vi "dummy VI.vi"   [LabVIEW 2020]
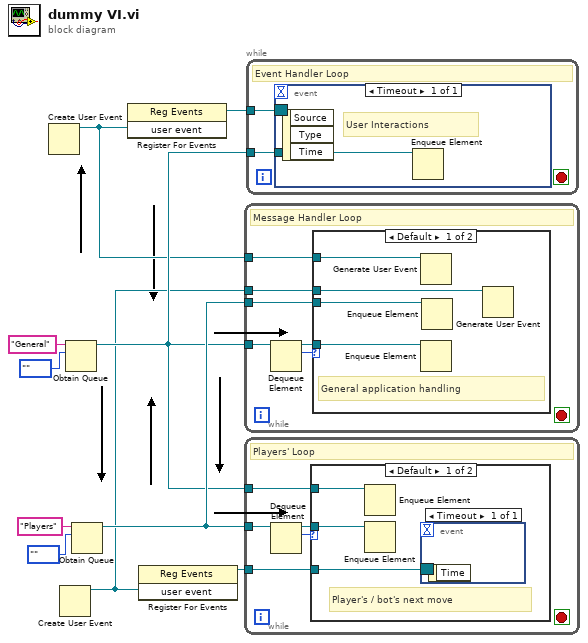
[diagram p0: block diagram]
diagram:
  n1 = Create User Event() -> (user event=w3:refnum<user-event>)  [unwired: 2 in, 1 out]
  n2 = Create User Event() -> (user event=w1:refnum<user-event>)  [unwired: 2 in, 1 out]
  n3 = Obtain Queue(name (unnamed)="General", element data type=enum16{""}."") -> (queue out=w7:refnum<queue>)  [unwired: 3 in, 2 out]
  n4 = Obtain Queue(name (unnamed)="Players", element data type=enum16{""}."") -> (queue out=w8:refnum<queue>)  [unwired: 3 in, 2 out]
  n5 = register-events(w3) -> (reference out=w4:refnum<event-registration>)  [unwired: 2 in, 1 out]
  n6 = register-events(w1) -> (reference out=w2:refnum<event-registration>)  [unwired: 2 in, 1 out]
  n7 = while {
    tunnel: w7 -> [w16]
    tunnel: w8 -> [w13]
    tunnel: w3 -> [w12]
    tunnel: w1 -> [w11]
    stop <- _ stop-if-true
    # "Message Handler Loop"
    n8 = Dequeue Element(queue=w16) -> (queue out=w14:refnum<queue>, element=w15:enum16{""})  [unwired: 2 in, 2 out]
    n9 = case shown="Default" w15 {
      tunnel: w14 -> [w20 _]
      tunnel: w13 -> [w19 _]
      tunnel: w12 -> [w18 _]
      tunnel: w11 -> [w17 _]
      frame Default {
        # "General application handling"
        n10 = Generate User Event(user event=w18) -> ()  [unwired: 3 in, 2 out]
        n11 = Enqueue Element(queue=w20) -> ()  [unwired: 3 in, 3 out]
        n12 = Enqueue Element(queue=w19) -> ()  [unwired: 3 in, 3 out]
        n13 = Generate User Event(user event=w17) -> ()  [unwired: 3 in, 2 out]
      }
      frame "" {
      }
    }
  }
  n14 = while {
    tunnel: w7 -> [w22]
    tunnel: w8 -> [w25]
    tunnel: w2 -> [w21]
    stop <- _ stop-if-true
    # "Players' Loop"
    n15 = Dequeue Element(queue=w25) -> (queue out=w23:refnum<queue>, element=w24:enum16{""})  [unwired: 2 in, 2 out]
    n16 = case shown="Default" w24 {
      tunnel: w23 -> [w27 _]
      tunnel: w22 -> [w28 _]
      tunnel: w21 -> [w26 _]
      frame #0 {
        # "Player's / bot's next move"
        n17 = Enqueue Element(queue=w28) -> ()  [unwired: 3 in, 3 out]
        n18 = Enqueue Element(queue=w27) -> ()  [unwired: 3 in, 3 out]
        n19 = event shown="[0] Timeout" {
          selector: w26 -> [_]
          dyn-events: _ -> [_]
          timeout: _ -> [_]
          event Timeout {
            n20 = event-data() -> ()  [unwired: 1 in, 1 out]
          }
        }
      }
      frame #1 {
      }
    }
  }
  n21 = while {
    tunnel: w7 -> [w29]
    tunnel: w4 -> [w30]
    stop <- _ stop-if-true
    # "Event Handler Loop"
    n22 = event shown="[0] Timeout" {
      selector: w30 -> [_]
      dyn-events: _ -> [_]
      timeout: _ -> [_]
      tunnel: w29 -> [w31]
      event Timeout {
        # "User Interactions"
        n23 = event-data() -> ()  [unwired: 1 in, 3 out]
        n24 = Enqueue Element(queue=w31) -> ()  [unwired: 3 in, 3 out]
      }
    }
  }
